vi "testIdxArrayToBoolArray.vi"(8 "error in (no error)":errorcluster) -> (0 "error out":errorcluster)   [LabVIEW 2016]
doc: "Test to translate the index array to boolean array."
uses:
  <vilib>/addons/_JKI Toolkits/Caraya/classes/Test/Test.lvclass
  <vilib>/addons/_JKI Toolkits/Caraya/classes/Assert/Assert.lvclass
  MatOper/MatOper.lvclass
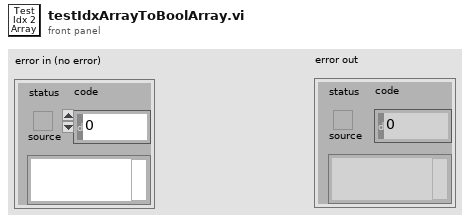
[diagram p1: front panel]
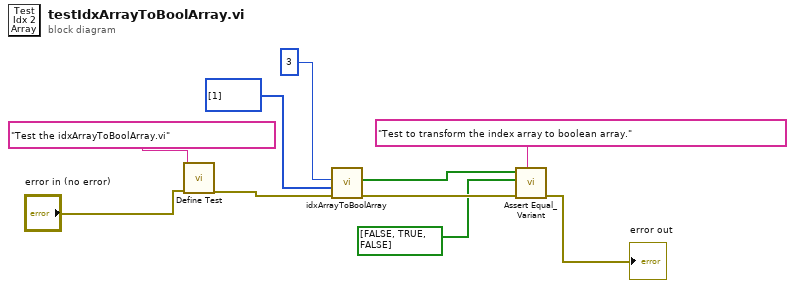
[diagram p0: block diagram]
diagram:
  n1 = call <vilib>:"Define Test.vi"("error in (no error)"="error in (no error)", "Label (VI Title)"="Test the idxArrayToBoolArray.vi") -> ("error out"=w6:errorcluster)  [unwired: 9 in]
  n2 = call "idxArrayToBoolArray.vi"("error in (no error)"=w6, "Idx Array"=i32[] [1], "Length of Bool Array"=3) -> ("error out"=w3:errorcluster, "Bool Array"=w2:bool[])  [unwired: 6 in, 1 out]
  n3 = call <vilib>:"Assert Equal_Variant.vi"("Label"="Test to transform the index array to boolean array.", "error in (no error)"=w3, "Y"=bool[] [FALSE, TRUE, FALSE] ("Bool Array"), "X"=w2) -> ("error out"=→"error out":errorcluster)  [unwired: 7 in]
